vi "SunplusDailyS2TAutoMultiplePart.vi"() -> ()   [LabVIEW 2012]
uses:
  <vilib>/addons/database/Auxilliary.llb/DB Tools Cursor Type.ctl
  <vilib>/Utility/NIReport.llb/NI_report.lvclass
  <vilib>/addons/database/Connection.llb/DB Tools Open Connec (Path).vi
  <vilib>/addons/database/Connection.llb/Conn Execute.vi
  <vilib>/addons/database/Recordset.llb/Rec Fetch Recordset Data (R).vi
  <vilib>/addons/database/Recordset.llb/Rec Destroy - Connection.vi
  <vilib>/addons/database/_DB Variant To Data/Database Variant To Data.xnode
  <vilib>/addons/database/NI_Database_API.lvlib
  <vilib>/Utility/SMTP/NI_SMTPEmail.lvlib
  <vilib>/Utility/NIReport.llb/Excel/NI_Excel.lvclass
panel:
  out "concatenated string":string
  in  "start (0, 0) 4":cluster{"start row":i32, "start column":i32}
  out "error out":errorcluster
  out "error out 2":errorcluster
  in  "MIME content-type (application/octet-stream)":string="application/octet-stream"
  out "error out 4":errorcluster
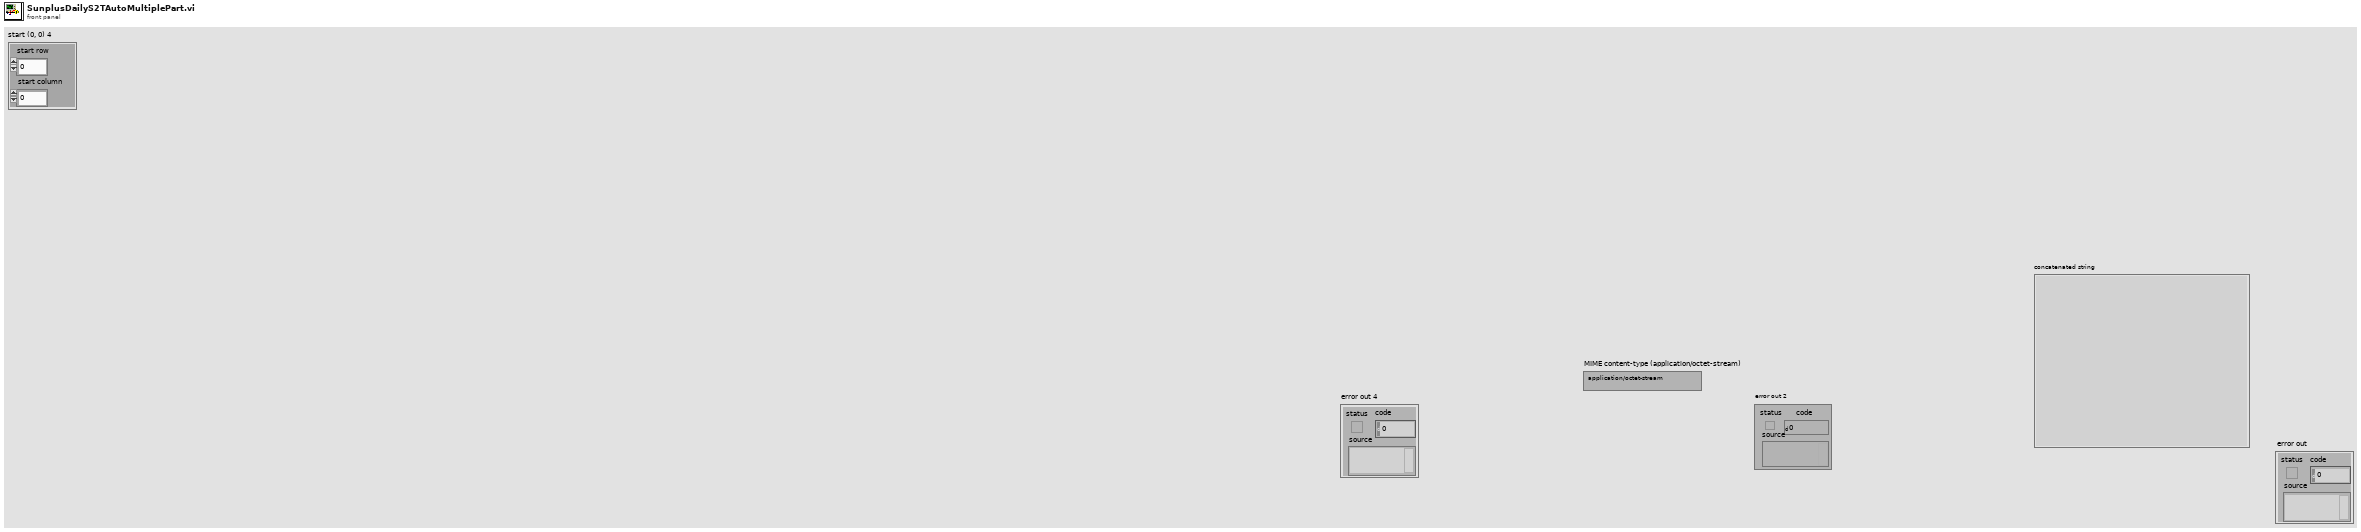
[diagram p1: front panel]
types:
  T1 = typedef "NI_Database_API.lvlib/DB Tools Cursor Type.ctl" = enum16{"forward-only", "keyset", "dynamic", "static"}
  T2 = enum16{"Standard Report", "HTML", "Word", "Excel"}
  T3 = typedef "NI_Database_API.lvlib/Conn ObjectReference.ctl" = refnum<k1>
  T4 = typedef "NI_Database_API.lvlib/Rec ObjectReference.ctl" = refnum<k1>
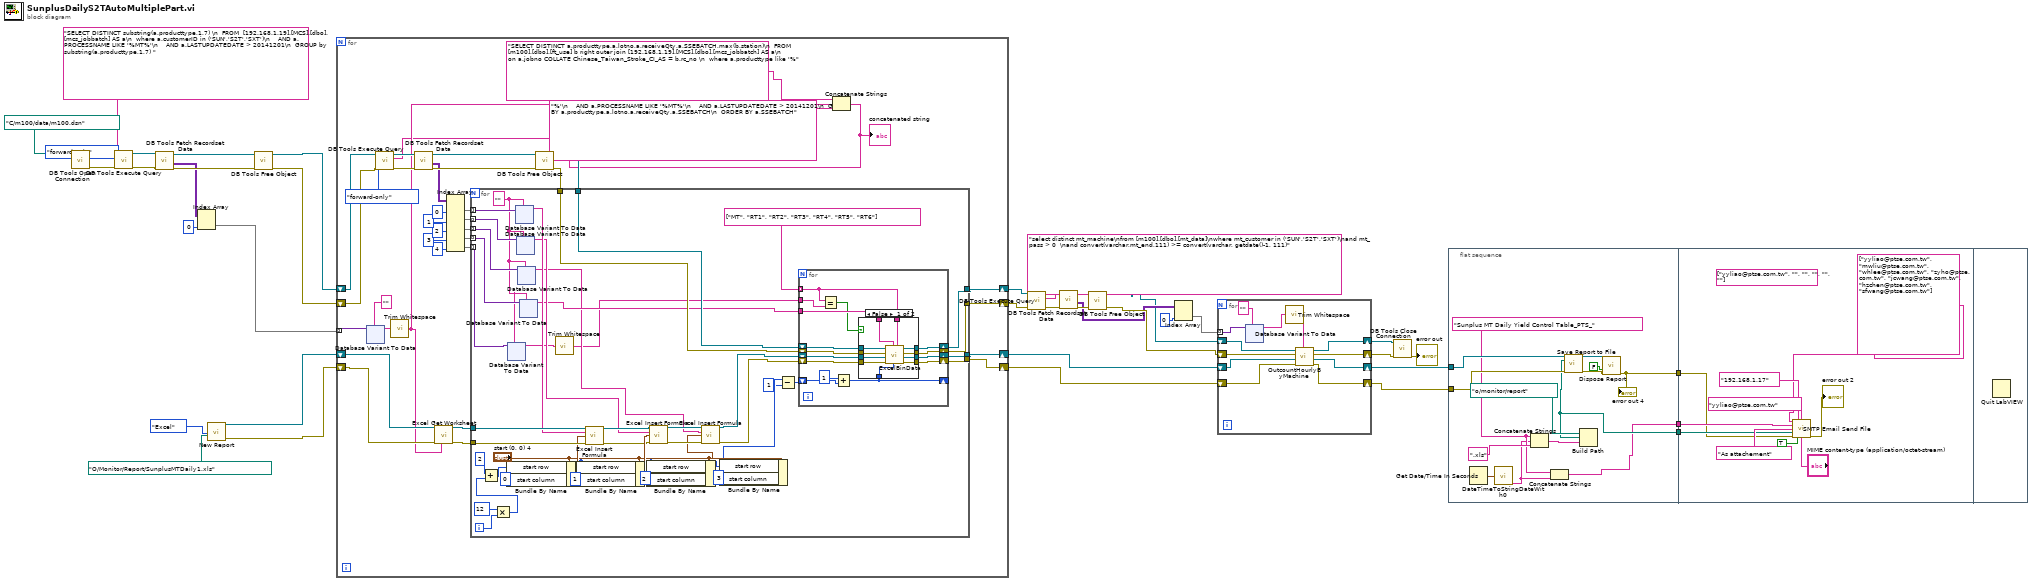
[diagram p0: block diagram]
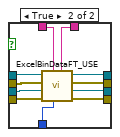
[diagram p2: hidden frame]
diagram:
  n1 = call-poly <vilib>:"DB Tools Open Connection.vi"("connection information"=path "C:/m100/data/m100.dsn") -> ("error out"=w24:errorcluster, "connection reference"=w25:T3)  [unwired: 7 in]
  n2 = call-poly <vilib>:"DB Tools Execute Query.vi"("error in (no error)"=w24, "cursor type"=DB_Tools_Cursor_Type."forward-only", "SQL query"="SELECT DISTINCT substring(a.producttype,1,7) \n  FROM  [192.168.1.19].[MCS].[dbo].[mcs_jobbatch] AS a\n  where a.customerID in ('SUN','S2T','SXT')\n    AND a.PROCESSNAME LIKE '%MT%'\n    AND a.LASTUPDATEDATE > 20141201\n  GROUP by substring(a.producttype,1,7) ", "connection reference"=w25) -> ("error out"=w22:errorcluster, "recordset reference"=w23:T4)  [unwired: 4 in]
  n3 = call-poly <vilib>:"DB Tools Fetch Recordset Data.vi"("error in (no error)"=w22, "recordset reference"=w23) -> ("error out"=w20:errorcluster, "recordset data"=w13:variant[][], "recordset reference out"=w21:T4)  [unwired: 3 in]
  n4 = Index Array(array=w13, index (col)=0 ("disabled index (col)")) -> (element=w11:variant[])  [unwired: 1 in]
  n5 = call <vilib>:"New Report.vi"("report type"=T2."Excel" ("Report Type"), "template (empty)"=path "O:/Monitor/Report/SunplusMTDaily1.xls") -> ("report out"=w15:refnum<class "NI_report.lvclass">, "error out"=w14:errorcluster)  [unwired: 12 in]
  n6 = call-poly <vilib>:"DB Tools Free Object.vi"("error in (no error)"=w20, "recordset reference"=w21) -> ("error out"=w16:errorcluster, "connection reference"=w17:T3)  [unwired: 8 in]
  n7 = for {
    shift-right: [w72] -> w7
    shift-left: w17 -> [w51]
    shift-right: [w73] -> w6
    shift-left: w16 -> [w50]
    shift-right: [w74] -> w26
    shift-left: w15 -> [w46]
    shift-right: [w75] -> w27
    shift-left: w14 -> [w45]
    tunnel: w11 -> [w49] mode=indexing
    n8 = xnode "Database Variant To Data"("database variant"=w49, "type"="") -> ("data"=w47:string)  [unwired: 1 in, 1 out]
    n9 = call <vilib>:"Trim Whitespace.vi"("string"=w47) -> ("trimmed string"=w43:string)  [unwired: 1 in]
    n10 = call <vilib>:"Excel Get Worksheet.vi"("report in"=w46, "error in (no error)"=w45, "name (\"\")"=w43) -> ("report out"=w55:refnum<class "NI_report.lvclass">, "error out"=w54:errorcluster)  [unwired: 11 in]
    n11 = Concatenate Strings("SELECT DISTINCT a.producttype,a.lotno,a.receiveQty,a.SSEBATCH,max(b.station)\n  FROM [m100].[dbo].[ft_use] b right outer join [192.168.1.19].[MCS].[dbo].[mcs_jobbatch] AS a\n  on a.jobno COLLATE Chinese_Taiwan_Stroke_CI_AS = b.rc_no \n  where a.producttype like '%" ("SQL query"), w43, "%'\n    AND a.PROCESSNAME LIKE '%MT%'\n    AND a.LASTUPDATEDATE > 20141201\n  GROUP BY a.producttype,a.lotno,a.receiveQty,a.SSEBATCH\n  ORDER BY a.SSEBATCH") -> (w41:string)
    "concatenated string" <- w41
    n12 = call-poly <vilib>:"DB Tools Execute Query.vi"("error in (no error)"=w50, "cursor type"=DB_Tools_Cursor_Type."forward-only", "SQL query"=w41, "connection reference"=w51) -> ("error out"=w68:errorcluster, "recordset reference"=w69:T4)  [unwired: 4 in]
    n13 = call-poly <vilib>:"DB Tools Fetch Recordset Data.vi"("error in (no error)"=w68, "recordset reference"=w69) -> ("error out"=w70:errorcluster, "recordset data"=w66:variant[][], "recordset reference out"=w71:T4)  [unwired: 3 in]
    n14 = Index Array(array=w66, index (col) #1=0 ("disabled index (col)"), index (col) #2=1 ("index (col)"), index (col) #3=2 ("index (col)"), index (col) #4=3 ("index (col)"), index (col) #5=4 ("index (col)")) -> (element #1=w62:variant[], element #2=w61:variant[], element #3=w60:variant[], element #4=w56:variant[], element #5=w52:variant[])  [unwired: 5 in]
    n15 = call-poly <vilib>:"DB Tools Free Object.vi"("error in (no error)"=w70, "recordset reference"=w71) -> ("error out"=w59:errorcluster, "connection reference"=w58:T3)  [unwired: 8 in]
    n16 = for {
      tunnel: w62 -> [w149] mode=indexing
      tunnel: w61 -> [w148] mode=indexing
      tunnel: w60 -> [w147] mode=indexing
      tunnel: w59 -> [w124]
      tunnel: w58 -> [w125]
      tunnel: w56 -> [w146] mode=indexing
      tunnel: w55 -> [w145]
      tunnel: w54 -> [w144]
      tunnel: [w115] -> w74
      tunnel: [w114] -> w75
      tunnel: [w117] -> w72
      tunnel: [w116] -> w73
      tunnel: w52 -> [w111] mode=indexing
      i -> [w128]
      w110 = ""
      n17 = Multiply(x=12, y=w128) -> (x*y=w126:i32)
      n18 = Add(x=2, y=w126) -> (x+y=w121:i32)
      n19 = Bundle By Name(cluster="start (0, 0) 4", "start row"=w121, "start column"=0) -> (w143:cluster{"start row":i32, "start column":i32})
      n20 = xnode "Database Variant To Data"("database variant"=w111, "type"=w110) -> ("data"=w109:string)  [unwired: 1 in, 1 out]
      n21 = xnode "Database Variant To Data"("database variant"=w149, "type"=w110) -> ("data"=w140:string)  [unwired: 1 in, 1 out]
      n22 = xnode "Database Variant To Data"("database variant"=w148, "type"=w110) -> ("data"=w135:string)  [unwired: 1 in, 1 out]
      n23 = xnode "Database Variant To Data"("database variant"=w147, "type"=w110) -> ("data"=w112:string)  [unwired: 1 in, 1 out]
      n24 = xnode "Database Variant To Data"("database variant"=w146, "type"=w110) -> ("data"=w118:string)  [unwired: 1 in, 1 out]
      n25 = call <vilib>:"Trim Whitespace.vi"("string"=w109) -> ("trimmed string"=w108:string)  [unwired: 1 in]
      n26 = Bundle By Name(cluster="start (0, 0) 4", "start row"=w121, "start column"=1) -> (w138:cluster{"start row":i32, "start column":i32})
      n27 = call <vilib>:"Excel Insert Formula.vi"("report in"=w145, "formula"=w140, "start (0, 0)"=w143, "error in (no error)"=w144) -> ("report out"=w137:refnum<class "NI_report.lvclass">, "error out"=w136:errorcluster)  [unwired: 10 in]
      n28 = Bundle By Name(cluster="start (0, 0) 4", "start row"=w121, "start column"=2) -> (w129:cluster{"start row":i32, "start column":i32})
      n29 = call <vilib>:"Excel Insert Formula.vi"("report in"=w137, "formula"=w135, "start (0, 0)"=w138, "error in (no error)"=w136) -> ("report out"=w133:refnum<class "NI_report.lvclass">, "error out"=w132:errorcluster)  [unwired: 10 in]
      n30 = call <vilib>:"Excel Insert Formula.vi"("report in"=w133, "formula"=w112, "start (0, 0)"=w129, "error in (no error)"=w132) -> ("report out"=w123:refnum<class "NI_report.lvclass">, "error out"=w122:errorcluster)  [unwired: 10 in]
      n31 = Bundle By Name(cluster="start (0, 0) 4", "start row"=w121, "start column"=3) -> ()  [unwired: 1 out]
      n32 = Subtract(x=w121, y=1) -> (x-y=w119:i32)
      n33 = for {
        shift-right: [w195] -> w117
        shift-left: w125 -> [w188]
        shift-right: [w194] -> w116
        shift-left: w124 -> [w187]
        shift-right: [w193] -> w115
        shift-left: w123 -> [w186]
        shift-right: [w192] -> w114
        shift-left: w122 -> [w185]
        shift-right: [w191] -> _
        shift-left: w119 -> [w190]
        tunnel: w118 -> [w189]
        tunnel: string[] ["MT", "RT1", "RT2", "RT3", "RT4", "RT5", "RT6"] ("Array") -> [w183] mode=indexing
        tunnel: w108 -> [w184]
        n34 = Equal?(x=w183, y=w184) -> (x = y?=w182:bool)
        n35 = Add(x=1, y=w190) -> (x+y=w191:i32)
        n36 = case shown="False" w182 {
          tunnel: [w207 w213] -> w195
          tunnel: [w206 w212] -> w194
          tunnel: [w205 w211] -> w193
          tunnel: [w204 w210] -> w192
          tunnel: w191 -> [w203 w218]
          tunnel: w189 -> [w202 w209]
          tunnel: w188 -> [w201 w217]
          tunnel: w187 -> [w200 w216]
          tunnel: w186 -> [w199 w215]
          tunnel: w185 -> [w198 w214]
          tunnel: w183 -> [w197 w208]
          frame False {
            n37 = call "ExcelBinData.vi"("step"=w197, "start row"=w203, "jobno"=w202, "error in (no error) 2"=w198, "report in"=w199, "error in (no error)"=w200, "connection reference 2"=w201) -> ("error out 2"=w204:errorcluster, "report out"=w205:refnum<class "NI_report.lvclass">, "error out"=w206:errorcluster, "connection reference"=w207:T3)  [unwired: 1 in]
          }
          frame True {
            n38 = call "ExcelBinDataFT_USE.vi"("step"=w208, "start row"=w218, "jobno"=w209, "error in (no error) 2"=w214, "report in"=w215, "error in (no error)"=w216, "connection reference 2"=w217) -> ("error out 2"=w210:errorcluster, "report out"=w211:refnum<class "NI_report.lvclass">, "error out"=w212:errorcluster, "connection reference"=w213:T3)  [unwired: 1 in]
          }
        }
      }
    }
  }
  n39 = call-poly <vilib>:"DB Tools Execute Query.vi"("error in (no error)"=w6, "SQL query"="select distinct mt_machine\nfrom [m100].[dbo].[mt_data]\nwhere mt_customer in ('SUN','S2T','SXT')\nand mt_pass > 0  \nand convert(varchar,mt_end,111) >= convert(varchar, getdate()-1, 111)", "connection reference"=w7) -> ("error out"=w10:errorcluster, "recordset reference"=w9:T4)  [unwired: 5 in]
  n40 = call-poly <vilib>:"DB Tools Fetch Recordset Data.vi"("error in (no error)"=w10, "recordset reference"=w9) -> ("error out"=w8:errorcluster, "recordset data"=w2:variant[][], "recordset reference out"=w5:T4)  [unwired: 3 in]
  n41 = call-poly <vilib>:"DB Tools Free Object.vi"("error in (no error)"=w8, "recordset reference"=w5) -> ("error out"=w3:errorcluster, "connection reference"=w1:T3)  [unwired: 8 in]
  n42 = Index Array(array=w2, index (col)=0 ("disabled index (col)")) -> (element=w34:variant[])  [unwired: 1 in]
  n43 = for {
    tunnel: w34 -> [w357] mode=indexing
    shift-right: [w352] -> w31
    shift-left: w1 -> [w350]
    shift-right: [w351] -> w30
    shift-left: w3 -> [w349]
    shift-right: [w355] -> w29
    shift-left: w26 -> [w358]
    shift-right: [w354] -> w28
    shift-left: w27 -> [w353]
    n44 = xnode "Database Variant To Data"("database variant"=w357, "type"="") -> ("data"=w348:string)  [unwired: 1 in, 1 out]
    n45 = call <vilib>:"Trim Whitespace.vi"("string"=w348) -> ("trimmed string"=w347:string)  [unwired: 1 in]
    n46 = call "OutcountHourlyByMachine.vi"("Machine"=w347, "error in (no error) 2"=w353, "report in"=w358, "error in (no error)"=w349, "connection reference"=w350) -> ("error in (no error) 3"=w354:errorcluster, "report in 2"=w355:refnum<class "NI_report.lvclass">, "error out"=w351:errorcluster, "connection reference 2"=w352:T3)  [unwired: 3 in]
  }
  n47 = call <vilib>:"DB Tools Close Connection.vi"("error in (no error)"=w30, "connection reference"=w31) -> ("error out"=→"error out":errorcluster)  [unwired: 5 in]
  n48 = flat-sequence {
    tunnel: w29 -> [w400]
    tunnel: w28 -> [w399]
    tunnel: [w391] -> w40
    tunnel: [w395] -> w39
    tunnel: [w394] -> w38
    tunnel: w40 -> [w408]
    tunnel: w39 -> [w407]
    tunnel: w38 -> [w406]
    frame #0 {
      w393 = "Sunplus MT Daily Yield Control Table_PTS_" ("string")
      n49 = Get Date/Time In Seconds() -> (seconds since 1Jan1904=w397:timestamp)
      n50 = call "DateTimeToStringDateWith0.vi"("time stamp"=w397) -> ("Dateyyyymmdd"=w392:string)  [unwired: 9 in, 1 out]
      n51 = Concatenate Strings(w393, w392, ".xls" ("string")) -> (w396:string)
      n52 = Concatenate Strings(w393, w392) -> (w391:string)
      n53 = Build Path(base path=path "o:/monitor/report", name or relative path=w396) -> (appended path=w395:path)
      n54 = call-dynamic "Save Report to File.vi"("report in"=w400, "report file path"=w395, "error in (no error)"=w399) -> ("report out"=w402:refnum<class "NI_report.lvclass">, "error out"=w401:errorcluster)  [unwired: 11 in]
      n55 = call-dynamic "Dispose Report.vi"("report in"=w402, "save changes? (F)"=FALSE, "error in (no error)"=w401) -> ("error out"=w394:errorcluster)  [unwired: 12 in]
      "error out 4" <- w394
    }
    frame #1 {
      (unwired) string[] ["yyliao@ptse.com.tw", "", "", "", "", ""] ("recipients")
      n56 = call <vilib>:"SMTP Email Send File.vi"("recipients"=string[] ["yyliao@ptse.com.tw", "mwliu@ptse.com.tw", "whlee@ptse.com.tw", "zyho@ptse.com.tw", "jcwang@ptse.com.tw", "hzchen@ptse.com.tw", "sfwang@ptse.com.tw"], "mail server"="192.168.1.17", "return address"="yyliao@ptse.com.tw", "subject ([No Subject])"=w408, "message"="As attachement", "file path"=w407, "error in (no error)"=w406, "binary? (F)"=TRUE, "MIME content-type (application/octet-stream)"="MIME content-type (application/octet-stream)") -> ("error out"=→"error out 2":errorcluster)  [unwired: 5 in, 1 out]
    }
    frame #2 {
      n57 = Quit LabVIEW() -> ()  [unwired: 1 in]
    }
  }
